vi "SendRaw.vi"() -> ()   [LabVIEW 2015]
uses:
  <vilib>/rvi/Emulation/niFpgaGetClockAttributes.vi
  <vilib>/rvi/Emulation/niFpgaSctlEmulationGetInTimedLoop.vi
  <vilib>/rvi/Emulation/niFpgaEmulationReportErrorSimple.vi
  <vilib>/rvi/DataTransferAndStorage/Container/Common/niFpgaContainerGetUniqueNameForEmu.vi
  <vilib>/rvi/DataTransferAndStorage/Container/Common/niFpgaContainerSetEmuInfo.vi
  <vilib>/rvi/eio/common/nirviEmuReportErrorAndStop.vi
  <vilib>/rvi/DataTransferAndStorage/Container/Common/niFpgaContainerExecOnDevCompGetState.vi
  <vilib>/rvi/Emulation/niFpgaEmulationIsFPGAContextNoSignature.vi
  <vilib>/rvi/errors/niFpgaSetErrorForExecOnDevCompSimple.vi
  <vilib>/rvi/FIFO/Fifo_Resource/nirvififoEmulationSetSize.vi
  <vilib>/rvi/FIFO/Fifo_Resource/nirviFifoEmulationQueueMgr.vi
  <instcachedir>/0/nirviFifoEmulationQueueMgr_E5CAEC123FF24DC58D834DCA3CDAA9B5.lvgen/nirviFifoEmulationQueueMgr_E5CAEC123FF24DC58D834DCA3CDAA9B5_002.vi
  <vilib>/rvi/FIFO/Fifo_Resource/nirvififoEmulationDetermineInputValidOut.vi
  <vilib>/rvi/FIFO/Fifo_Resource/nirvififoEmulationCreateLock.vi
  <vilib>/rvi/Emulation/niFpgaProcessEmulError.vi
  <vilib>/rvi/FIFO/Fifo_Resource/nirvififoEmulationObtainLock.vi
  <vilib>/rvi/FIFO/Fifo_Resource/nirvififoEmulationReleaseLock.vi
  <vilib>/rvi/occurrence/nirviWaitOnOccurrenceBase.vi
  <vilib>/rvi/errors/nirviReportUnexpectedCaseInternalError.vi
  <vilib>/rvi/errors/nirviReportUnexpectedCaseInternalError (U32).vi
  <vilib>/Utility/error.llb/Clear Errors.vi
  <vilib>/rvi/interface/RandomDataEmulation/niFpgaRandomDataHandleErrors.vi
  <vilib>/rvi/Emulation/niFpgaCriticalErrorInLSC.vi
  <instcachedir>/0/nirviFifoEmulationQueueMgr_E5CAEC123FF24DC58D834DCA3CDAA9B5.lvgen/nirviFifoEmulationQueueMgr_E5CAEC123FF24DC58D834DCA3CDAA9B5_008.vi
  <vilib>/rvi/eio/common/nirviEmuTemplateMethod_errors.vi
  <vilib>/rvi/LocalResourceManager/LocalResourceManager.xnode
  <vilib>/rvi/DataTransferAndStorage/Container/XNode/niFpgaContainer.xnode
  <vilib>/rvi/FIFO/Fifo_Resource/niFpgaFifoEmulationRefIn.vi
  <vilib>/rvi/interface/RandomDataEmulation/nirviRandomDataFpgaReadWriteTemplate.vi
  <vilib>/eio/EIONode/EIONode.xnode
panel:
  out "Max Correlation 3":fxp<+/-,33,17> format="%.22g"
  out "TDOA 3":u16
  out "Trigger 3":bool
  out "Max Correlation 2":fxp<+/-,33,17> format="%.22g"
  out "TDOA 2":u16
  out "Trigger 2":bool
  out "Max Correlation 1":fxp<+/-,33,17> format="%.22g"
  out "TDOA 1":u16
  out "Trigger 1":bool
  out "Cross Correlation 3":fxp<+/-,32,16>
  out "Cross Correlation 2":fxp<+/-,32,16>
  out "Cross Correlation 1":fxp<+/-,32,16>
  in  "Baud Rate":u32=9600
  out "Raw 3":fxp<+/-,16,4> format="%.24g"
  out "Raw 2":fxp<+/-,16,4> format="%.24g"
  out "Raw 1":fxp<+/-,16,4> format="%.24g"
  out "Raw 0":fxp<+/-,16,4> format="%.24g"
  in  "Input period (ticks)":i16=80
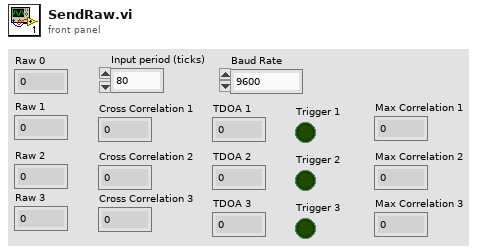
[diagram p1: front panel]
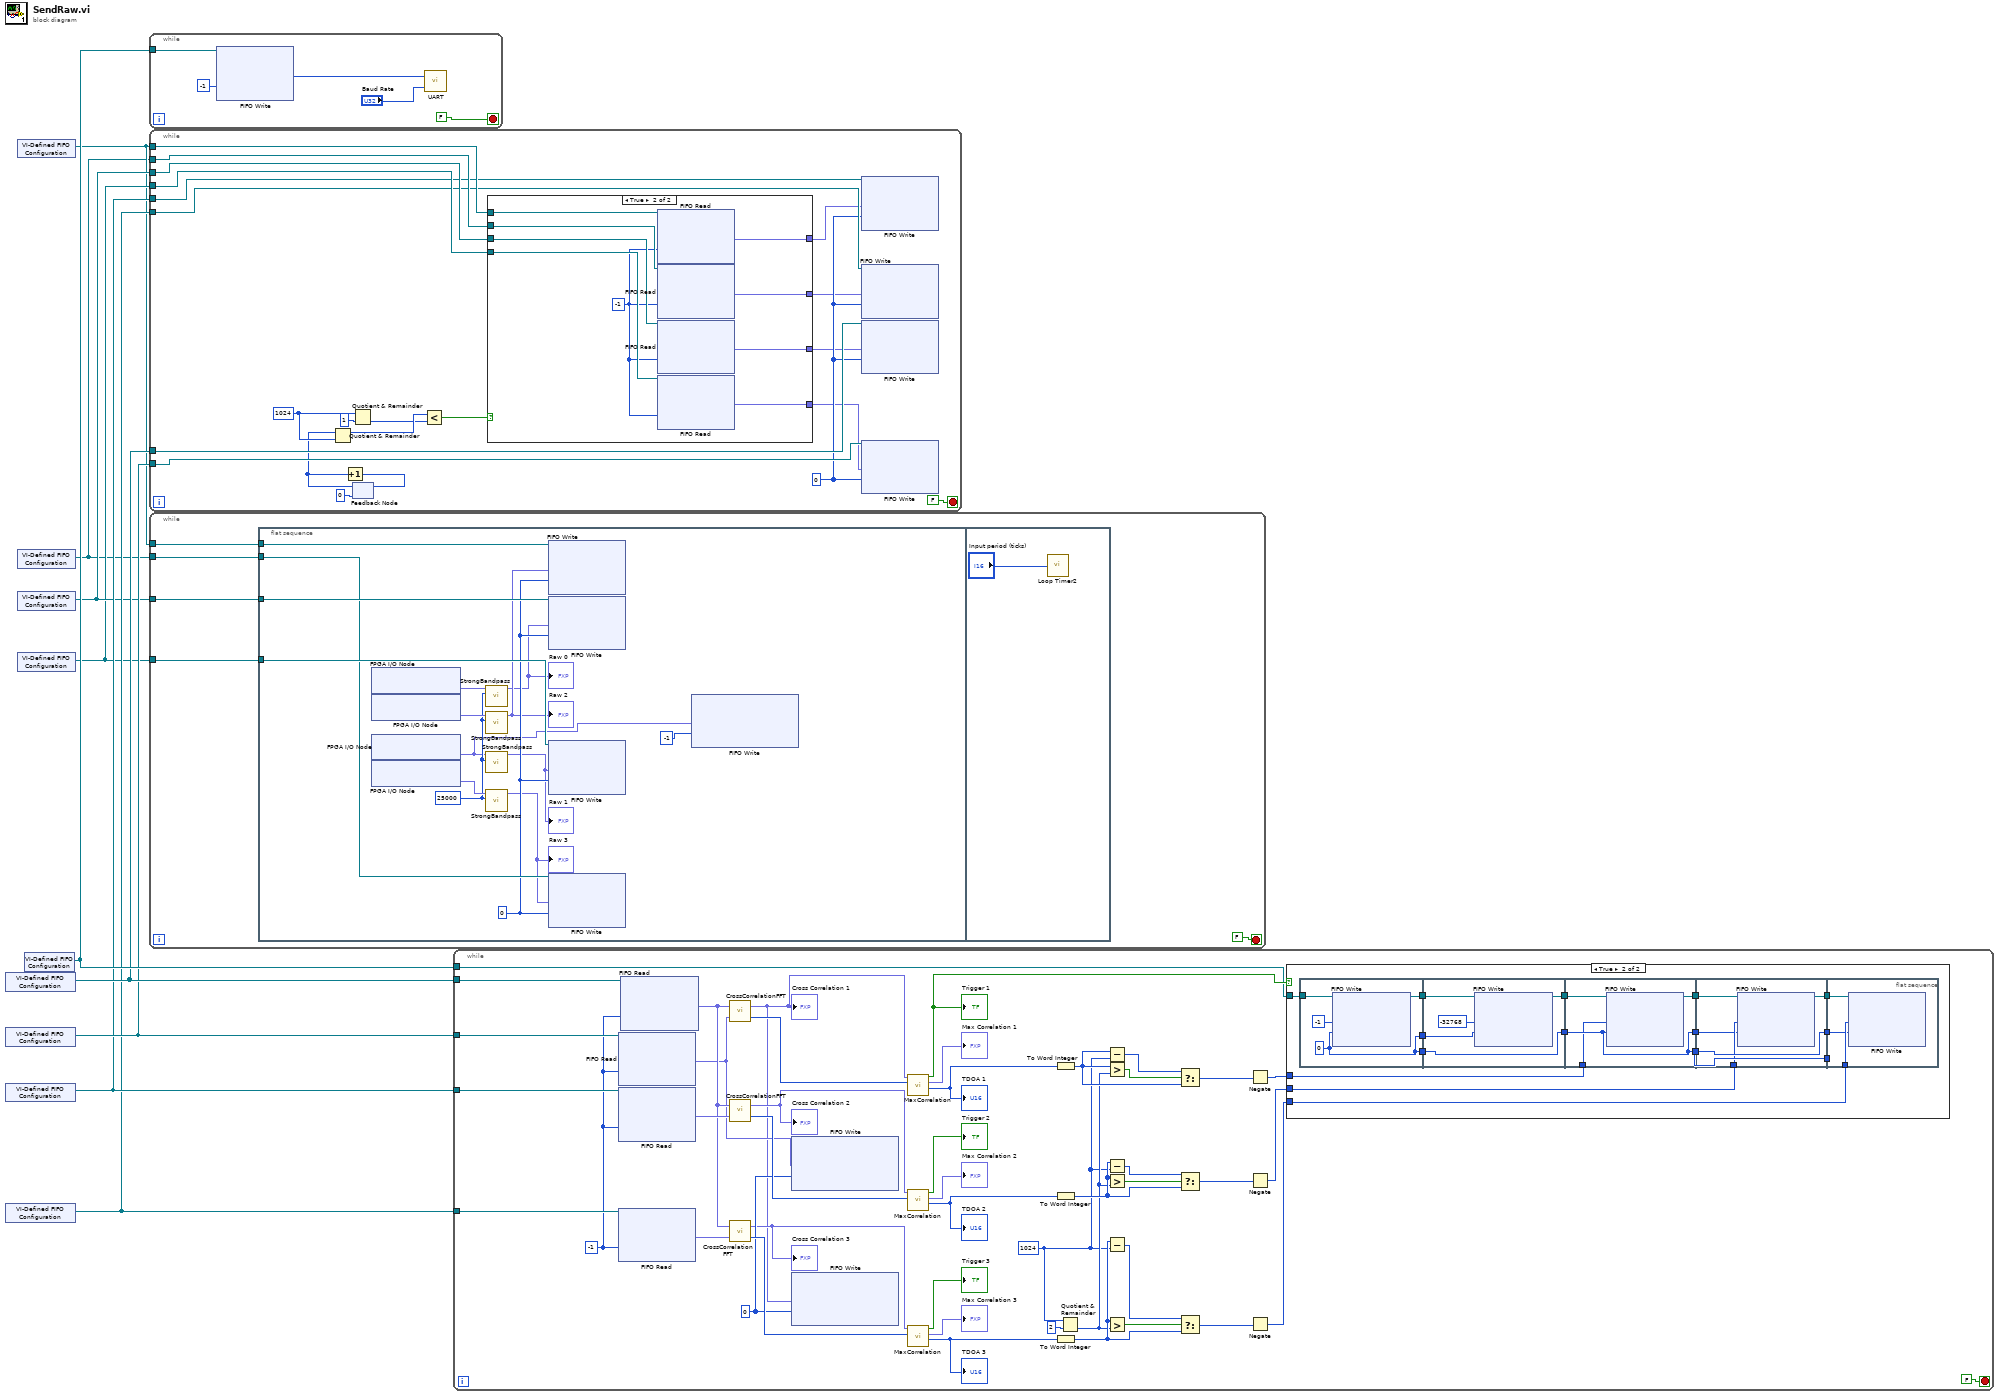
[diagram p0: block diagram]
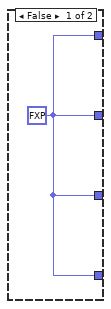
[diagram p3: hidden frame]
diagram:
  n1 = xnode "VI-Defined FIFO Configuration"() -> ("FIFO Out"=w8:refnum<k21>)
  n2 = xnode "VI-Defined FIFO Configuration"() -> ("FIFO Out"=w7:refnum<k21>)
  n3 = xnode "VI-Defined FIFO Configuration"() -> ("FIFO Out"=w6:refnum<k21>)
  n4 = xnode "VI-Defined FIFO Configuration"() -> ("FIFO Out"=w5:refnum<k21>)
  n5 = xnode "VI-Defined FIFO Configuration"() -> ("FIFO Out"=w2:refnum<k21>)
  n6 = xnode "VI-Defined FIFO Configuration"() -> ("FIFO Out"=w1:refnum<k21>)
  n7 = xnode "VI-Defined FIFO Configuration"() -> ("FIFO Out"=w4:refnum<k21>)
  n8 = xnode "VI-Defined FIFO Configuration"() -> ("FIFO Out"=w3:refnum<k21>)
  n9 = xnode "VI-Defined FIFO Configuration"() -> ("FIFO Out"=w9:refnum<k21>)
  n10 = while {
    tunnel: w9 -> [w14]
    stop <- FALSE stop-if-true
    n11 = xnode ("FIFO Write")("Timeout"=i16 -1, "FIFO In"=w14) -> ("Element"=w11:i16)  [unwired: 2 out]
    n12 = call "UART.vi"("Baud Rate"="Baud Rate", "Input"=w11) -> ()  [unwired: 1 in]
  }
  n13 = while {
    tunnel: w4 -> [w31]
    tunnel: w3 -> [w29]
    tunnel: w2 -> [w30]
    tunnel: w1 -> [w28]
    tunnel: w8 -> [w27]
    tunnel: w7 -> [w26]
    tunnel: w6 -> [w25]
    tunnel: w5 -> [w24]
    stop <- FALSE stop-if-true
    w23 = i16 0
    w35 = i16 1024
    n14 = Quotient & Remainder(x=w35, y=i16 1) -> (floor(x/y)=w15:i16)  [unwired: 1 out]
    n15 = feedback #1(u64 0) -> (w16:u64)
    n16 = Quotient & Remainder(x=w16, y=w35) -> (x-y*floor(x/y)=w33:u64)  [unwired: 1 out]
    n17 = Increment(x=w16) -> (x+1=w18:u64)
    n18 = feedback-in #1(w18) -> ()
    n19 = Less?(x=w33, y=w15) -> (x < y?=w32:bool)
    n20 = case shown="True" w32 {
      tunnel: w31 -> [_ w46]
      tunnel: w29 -> [_ w45]
      tunnel: w30 -> [_ w44]
      tunnel: w28 -> [_ w43]
      tunnel: [w37 w41] -> w22
      tunnel: [w37 w40] -> w21
      tunnel: [w37 w39] -> w20
      tunnel: [w37 w38] -> w19
      frame False {
        w37 = fxp<+/-,32,16> 0.0
      }
      frame True {
        w42 = i16 -1
        n21 = xnode ("FIFO Read")("Timeout"=w42, "FIFO In"=w44) -> ("Element"=w41:fxp<+/-,32,16>)  [unwired: 2 out]
        n22 = xnode ("FIFO Read")("Timeout"=w42, "FIFO In"=w43) -> ("Element"=w40:fxp<+/-,32,16>)  [unwired: 2 out]
        n23 = xnode ("FIFO Read")("Timeout"=w42, "FIFO In"=w46) -> ("Element"=w38:fxp<+/-,32,16>)  [unwired: 2 out]
        n24 = xnode ("FIFO Read")("Timeout"=w42, "FIFO In"=w45) -> ("Element"=w39:fxp<+/-,32,16>)  [unwired: 2 out]
      }
    }
    n25 = xnode ("FIFO Write")("Element"=w22, "Timeout"=w23, "FIFO In"=w25) -> ()  [unwired: 2 out]
    n26 = xnode ("FIFO Write")("Element"=w21, "Timeout"=w23, "FIFO In"=w24) -> ()  [unwired: 2 out]
    n27 = xnode ("FIFO Write")("Element"=w19, "Timeout"=w23, "FIFO In"=w27) -> ()  [unwired: 2 out]
    n28 = xnode ("FIFO Write")("Element"=w20, "Timeout"=w23, "FIFO In"=w26) -> ()  [unwired: 2 out]
  }
  n29 = while {
    tunnel: w4 -> [w50]
    tunnel: w3 -> [w49]
    tunnel: w2 -> [w48]
    tunnel: w1 -> [w47]
    stop <- FALSE stop-if-true
    n30 = flat-sequence {
      tunnel: w50 -> [w62]
      tunnel: w49 -> [w61]
      tunnel: w48 -> [w60]
      tunnel: w47 -> [w59]
      frame #0 {
        w58 = i16 0
        w63 = 25000
        n31 = xnode "FPGA I/O Node"() -> ("Connector0/AI0"=w66:fxp<+/-,27,5>)  [unwired: 1 in, 1 out]
        n32 = xnode "FPGA I/O Node"() -> ("Connector0/AI2"=w65:fxp<+/-,27,5>)  [unwired: 1 in, 1 out]
        n33 = xnode "FPGA I/O Node"() -> ("Connector0/AI1"=w53:fxp<+/-,27,5>)  [unwired: 1 in, 1 out]
        n34 = xnode "FPGA I/O Node"() -> ("Connector0/AI3"=w64:fxp<+/-,27,5>)  [unwired: 1 in, 1 out]
        n35 = call "StrongBandpass.vi"("Frequency"=w63, "Numeric"=w66) -> ("Output"=w55:fxp<+/-,16,4>)  [unwired: 9 in]
        "Raw 0" <- w55
        n36 = call "StrongBandpass.vi"("Frequency"=w63, "Numeric"=w65) -> ("Output"=w56:fxp<+/-,16,4>)  [unwired: 9 in]
        "Raw 2" <- w56
        n37 = call "StrongBandpass.vi"("Frequency"=w63, "Numeric"=w53) -> ("Output"=w54:fxp<+/-,16,4>)  [unwired: 9 in]
        "Raw 1" <- w54
        n38 = call "StrongBandpass.vi"("Frequency"=w63, "Numeric"=w64) -> ("Output"=w57:fxp<+/-,16,4>)  [unwired: 9 in]
        "Raw 3" <- w57
        n39 = xnode ("FIFO Write")("Element"=w56, "Timeout"=w58, "FIFO In"=w60) -> ()  [unwired: 2 out]
        n40 = xnode ("FIFO Write")("Element"=w55, "Timeout"=w58, "FIFO In"=w62) -> ()  [unwired: 2 out]
        n41 = xnode ("FIFO Write")("Element"=w54, "Timeout"=w58, "FIFO In"=w61) -> ()  [unwired: 2 out]
        n42 = xnode ("FIFO Write")("Element"=w57, "Timeout"=w58, "FIFO In"=w59) -> ()  [unwired: 2 out]
        n43 = xnode ("FIFO Write")("Element"=w53, "Timeout"=i16 -1) -> ()  [unwired: 1 in, 2 out]
      }
      frame #1 {
        n44 = call "Loop Timer2"("Count(Ticks)"="Input period (ticks)") -> ()  [unwired: 1 out]
      }
    }
  }
  n45 = while {
    tunnel: w8 -> [w100]
    tunnel: w7 -> [w99]
    tunnel: w6 -> [w98]
    tunnel: w5 -> [w97]
    tunnel: w9 -> [w93]
    stop <- FALSE stop-if-true
    w71 = i16 1024
    w92 = i16 -1
    w104 = i16 0
    n46 = xnode ("FIFO Read")("Timeout"=w92, "FIFO In"=w99) -> ("Element"=w70:fxp<+/-,32,16>)  [unwired: 2 out]
    n47 = xnode ("FIFO Read")("Timeout"=w92, "FIFO In"=w98) -> ("Element"=w96:fxp<+/-,32,16>)  [unwired: 2 out]
    n48 = xnode ("FIFO Read")("Timeout"=w92, "FIFO In"=w97) -> ("Element"=w94:fxp<+/-,32,16>)  [unwired: 2 out]
    n49 = xnode ("FIFO Read")("Timeout"=w92, "FIFO In"=w100) -> ("Element"=w95:fxp<+/-,32,16>)  [unwired: 2 out]
    n50 = call "CrossCorrelationFFT.vi"("Input 2"=w70, "Input 1"=w95) -> ("Index"=w69:u16, "Cross Correlation"=w68:fxp<+/-,32,16>)
    "Cross Correlation 1" <- w68
    n51 = call "CrossCorrelationFFT.vi"("Input 2"=w96, "Input 1"=w95) -> ("Index"=w105:u16, "Cross Correlation"=w102:fxp<+/-,32,16>)
    "Cross Correlation 2" <- w102
    n52 = call "CrossCorrelationFFT.vi"("Input 2"=w94, "Input 1"=w95) -> ("Index"=w106:u16, "Cross Correlation"=w103:fxp<+/-,32,16>)
    "Cross Correlation 3" <- w103
    n53 = xnode ("FIFO Write")("Element"=w70, "Timeout"=w104) -> ()  [unwired: 1 in, 2 out]
    n54 = xnode ("FIFO Write")("Element"=w68, "Timeout"=w104) -> ()  [unwired: 1 in, 2 out]
    n55 = call "MaxCorrelation.vi"("Index in"=w69, "Cross Correlation"=w68) -> ("Index out"=w79:u16, "Numeric"=→"Max Correlation 1":fxp<+/-,33,17>, "Boolean"=w101:bool)  [unwired: 7 in]
    "Trigger 1" <- w101
    "TDOA 1" <- w79
    n56 = call "MaxCorrelation.vi"("Index in"=w105, "Cross Correlation"=w102) -> ("Index out"=w77:u16, "Numeric"=→"Max Correlation 2":fxp<+/-,33,17>, "Boolean"=→"Trigger 2":bool)  [unwired: 7 in]
    "TDOA 2" <- w77
    n57 = call "MaxCorrelation.vi"("Index in"=w106, "Cross Correlation"=w103) -> ("Index out"=w75:u16, "Numeric"=→"Max Correlation 3":fxp<+/-,33,17>, "Boolean"=→"Trigger 3":bool)  [unwired: 7 in]
    "TDOA 3" <- w75
    n58 = To Word Integer(number=w79) -> (16bit integer=w88:i16)
    n59 = To Word Integer(number=w77) -> (16bit integer=w84:i16)
    n60 = To Word Integer(number=w75) -> (16bit integer=w80:i16)
    n61 = Quotient & Remainder(x=w71, y=i16 2) -> (floor(x/y)=w72:i16)  [unwired: 1 out]
    n62 = Subtract(x=w88, y=w71) -> (x-y=w91:i16)
    n63 = Greater?(x=w88, y=w72) -> (0:w90:bool)
    n64 = Subtract(x=w84, y=w71) -> (x-y=w87:i16)
    n65 = Greater?(x=w84, y=w72) -> (0:w86:bool)
    n66 = Subtract(x=w80, y=w71) -> (x-y=w83:i16)
    n67 = Greater?(x=w80, y=w72) -> (0:w82:bool)
    n68 = Select(t=w91, s=w90, f=w88) -> (s? t:f=w89:i16)
    n69 = Select(t=w87, s=w86, f=w84) -> (s? t:f=w85:i16)
    n70 = Select(t=w83, s=w82, f=w80) -> (s? t:f=w81:i16)
    n71 = Negate(x=w89) -> (-x=w78:i16)
    n72 = Negate(x=w85) -> (-x=w76:i16)
    n73 = Negate(x=w81) -> (-x=w74:i16)
    n74 = case shown="True" w101 {
      tunnel: w78 -> [_ w113]
      tunnel: w76 -> [_ w116]
      tunnel: w74 -> [_ w115]
      tunnel: w93 -> [_ w114]
      frame False {
      }
      frame True {
        n75 = flat-sequence {
          tunnel: [w128] -> w127
          tunnel: w114 -> [w130]
          tunnel: [w129] -> w126
          tunnel: [w128] -> w125
          tunnel: w127 -> [w136]
          tunnel: [w136] -> w124
          tunnel: w126 -> [w135]
          tunnel: [w134] -> w123
          tunnel: w125 -> [w133]
          tunnel: [w140] -> w122
          tunnel: [w140] -> w121
          tunnel: [w138] -> w120
          tunnel: w124 -> [w140]
          tunnel: w123 -> [w139]
          tunnel: w113 -> [w137]
          tunnel: w122 -> [w141]
          tunnel: [w145] -> w119
          tunnel: w121 -> [w145]
          tunnel: [w145] -> w118
          tunnel: w116 -> [w142]
          tunnel: w120 -> [w144]
          tunnel: [w143] -> w117
          tunnel: w119 -> [w146]
          tunnel: w118 -> [_]
          tunnel: w115 -> [w147]
          tunnel: w117 -> [w148]
          frame #0 {
            w128 = i16 0
            n76 = xnode ("FIFO Write")("Element"=i16 -1, "Timeout"=w128, "FIFO In"=w130) -> ("FIFO Out"=w129:refnum<k21>)  [unwired: 1 out]
          }
          frame #1 {
            n77 = xnode ("FIFO Write")("Element"=i16 -32768, "Timeout"=w133, "FIFO In"=w135) -> ("FIFO Out"=w134:refnum<k21>)  [unwired: 1 out]
          }
          frame #2 {
            n78 = xnode ("FIFO Write")("Element"=w137, "Timeout"=w140, "FIFO In"=w139) -> ("FIFO Out"=w138:refnum<k21>)  [unwired: 1 out]
          }
          frame #3 {
            n79 = xnode ("FIFO Write")("Element"=w142, "Timeout"=w141, "FIFO In"=w144) -> ("FIFO Out"=w143:refnum<k21>)  [unwired: 1 out]
          }
          frame #4 {
            n80 = xnode ("FIFO Write")("Element"=w147, "Timeout"=w146, "FIFO In"=w148) -> ()  [unwired: 2 out]
          }
        }
      }
    }
  }
